vi "N channel N  sample API( data reading).vi"() -> ()   [LabVIEW 2020]
uses:
  <vilib>/DAQmx/read.llb/DAQmx Read (Analog 2D DBL NChan NSamp).vi
  <vilib>/DAQmx/create/channels.llb/DAQmx Create Channel (AI-Temperature-Thermocouple).vi
  <vilib>/DAQmx/configure/timing.llb/DAQmx Timing (Sample Clock).vi
  <vilib>/DAQmx/miscellaneous.llb/DAQmx Fill In Error Info.vi
panel:
  out "Waveform Graph":dbl[][](graph)
  in  "number of samples per channel( user defined to read from the daq)":i32=-1
  out "Array":dbl[][](array[numeric]) format="%0.2f"
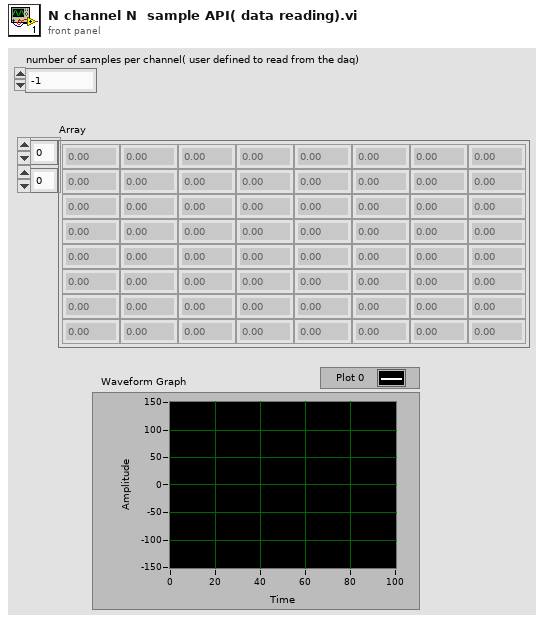
[diagram p1: front panel]
types:
  T1 = enum16{"open", "replace", "create", "open or create", "replace or create", "replace or create with confirmation"}
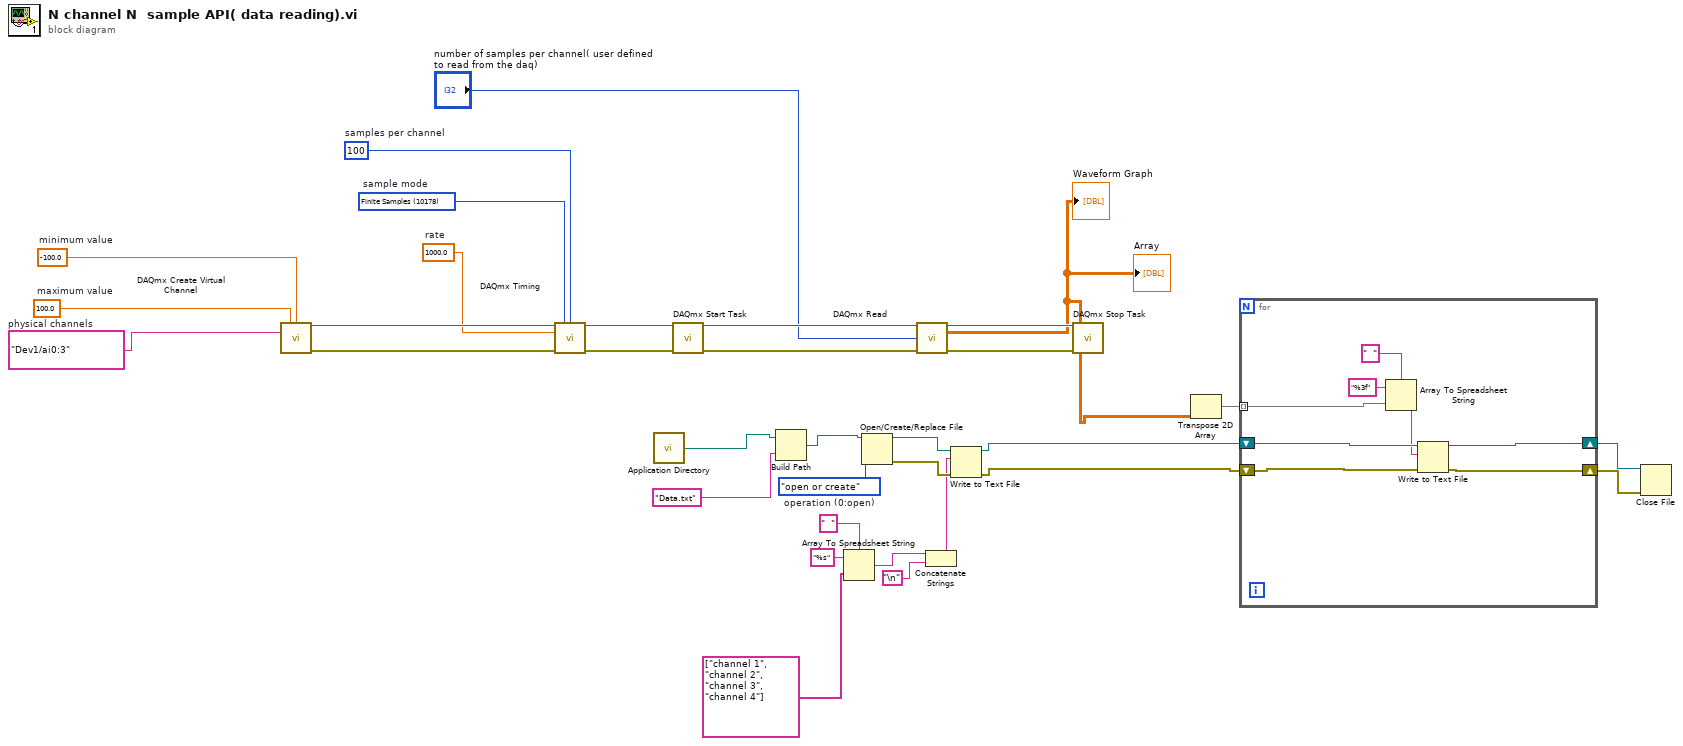
[diagram p0: block diagram]
diagram:
  w15 = T1."open or create"  # operation (0:open)
  w20 = 1000.0  # rate
  w23 = 10178 items=["Finite Samples"=10178, "Continuous Samples"=10123, "Hardware Timed Single Point"=12522]  # sample mode
  w24 = 100  # samples per channel
  w25 = 100.0  # maximum value
  w26 = -100.0  # minimum value
  w27 = tag "Dev1/ai0:3"  # physical channels
  n1 = call-poly <vilib>:"DAQmx Create Virtual Channel.vi"("maximum value"=w25, "minimum value"=w26, "physical channels"=w27) -> ("task out"=w22:refnum<k21>, "error out"=w31:errorcluster)  [unwired: 11 in]
  n2 = call-poly <vilib>:"DAQmx Timing.vi"("task/channels in"=w22, "sample mode"=w23, "samples per channel"=w24, "rate"=w20, "error in"=w31) -> ("task out"=w21:refnum<k21>, "error out"=w30:errorcluster)  [unwired: 9 in]
  n3 = call <vilib>:"Application Directory.vi"() -> ("Application Directory"=w18:path)
  n4 = call <vilib>:"DAQmx Start Task.vi"("task/channels in"=w21, "error in"=w30) -> ("task out"=w33:refnum<k21>, "error out"=w29:errorcluster)  [unwired: 12 in]
  n5 = Build Path(base path=w18, name or relative path="Data.txt") -> (appended path=w16:path)
  n6 = Array To Spreadsheet String(delimiter (Tab)="  ", array=string[] ["channel 1", "channel 2", "channel 3", "channel 4"], 3:"%s" ("format string")) -> (spreadsheet string=w3:string)
  n7 = Open/Create/Replace File(file path (use dialog)=w16, operation (0:open)=w15) -> (refnum out=w14:refnum<file>, error out=w13:errorcluster)  [unwired: 4 in, 1 out]
  n8 = call-poly <vilib>:"DAQmx Read.vi"("task/channels in"=w33, "number of samples per channel"="number of samples per channel( user defined to read from the daq)", "error in"=w29) -> ("task out"=w32:refnum<k21>, "data"=w9:dbl[][], "error out"=w28:errorcluster)  [unwired: 10 in]
  "Array" <- w9
  "Waveform Graph" <- w9
  n9 = Concatenate Strings(w3, "\n") -> (w1:string)
  n10 = Write to Text File(file (use dialog)=w14, text=w1, error in=w13) -> (refnum out=w10:refnum<file>, error out=w7:errorcluster)  [unwired: 1 in, 1 out]
  n11 = call <vilib>:"DAQmx Stop Task.vi"("task/channels in"=w32, "error in"=w28) -> ()  [unwired: 12 in, 2 out]
  n12 = Transpose 2D Array(2D array=w9) -> (transposed array=w8:dbl[][])
  n13 = for {
    shift-right: [w40] -> w11
    shift-left: w10 -> [w39]
    tunnel: w8 -> [w38] mode=indexing
    shift-right: [w41] -> w12
    shift-left: w7 -> [w35]
    n14 = Array To Spreadsheet String(delimiter (Tab)="  ", array=w38, 3:"%3f" ("format string")) -> (spreadsheet string=w34:string)
    n15 = Write to Text File(file (use dialog)=w39, text=w34, error in=w35) -> (refnum out=w40:refnum<file>, error out=w41:errorcluster)  [unwired: 1 in, 1 out]
  }
  n16 = Close File(refnum=w11, error in=w12) -> ()  [unwired: 2 out]
